vi "Motor Adjustment.vi"(9 "Offset":dbl(knob) scale=0.0..1.0, 10 "Dead Zone":dbl(knob) scale=0.0..1.0, 11 "X in":dbl) -> (3 "X Out":dbl)   [LabVIEW 2015]
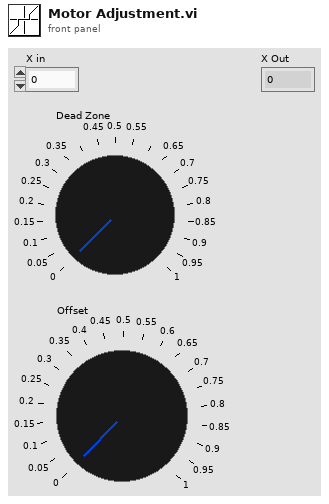
[diagram p1: front panel]
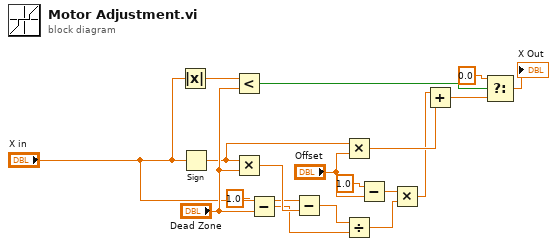
[diagram p0: block diagram]
diagram:
  n1 = Absolute Value(x="X in") -> (abs(x)=w1:dbl)
  n2 = Sign(1:"X in") -> (0:w16:dbl)
  n3 = Less?(x=w1, y="Dead Zone") -> (x < y?=w2:bool)
  n4 = Multiply(x=w16, y="Dead Zone") -> (x*y=w18:dbl)
  n5 = Subtract(x=1.0, y="Dead Zone") -> (x-y=w4:dbl)
  n6 = Subtract(x="X in", y=w18) -> (x-y=w15:dbl)
  n7 = Multiply(x=w16, y="Offset") -> (x*y=w13:dbl)
  n8 = Divide(x=w15, y=w4) -> (x/y=w6:dbl)
  n9 = Subtract(x=1.0, y="Offset") -> (x-y=w8:dbl)
  n10 = Multiply(x=w8, y=w6) -> (x*y=w9:dbl)
  n11 = Add(x=w9, y=w13) -> (x+y=w10:dbl)
  n12 = Select(t=0.0, s=w2, f=w10) -> (s? t:f=→"X Out":dbl)
